vi "WaveformDataEventHandler Event Callback (CDB).vi"(4 "user event":refnum<user-event>, 5 "Event Data":cluster{"sender":refnum<k24>, "e":refnum<k24>}, 6 "Control Ref":refnum<k24>, 7 "Event Common Data":T1) -> ()   [LabVIEW 2020, in "NI_VS Waveform Streaming Interface.lvlib"]
uses:
  <vilib>/NI VeriStand/Execution/WaveformStreaming/NI_VS Waveform Streaming Interface.lvlib
  NationalInstruments.VeriStand.ClientAPI
  <vilib>/NI VeriStand/Execution/WaveformStreaming/Waveform Data Watcher Event Data (CDB).ctl
  <vilib>/NI VeriStand/Execution/WaveformStreaming/WaveformStreamSpecification.ctl
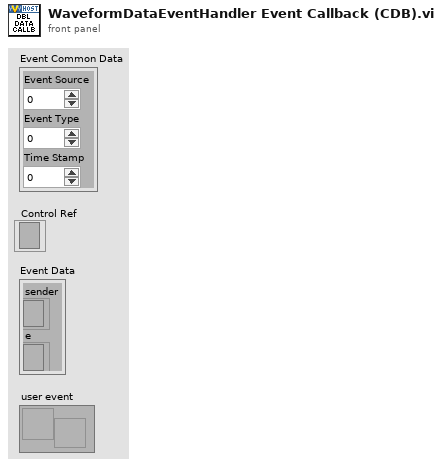
[diagram p1: front panel]
types:
  T1 = cluster{"Event Source":i32, "Event Type":u32, "Time Stamp":u32}
  T2 = typedef "NI_VS Waveform Streaming Interface.lvlib/Waveform Data Watcher Event Data (CDB).ctl" = cluster{"Data":cdb[], "dt":dbl, "offset from start (samples)":u64, "t0 at start":timestamp, "WaveformStreamSpecification":T3}
  T3 = typedef "NI_VS Waveform Streaming Interface.lvlib/WaveformStreamSpecification.ctl" = refnum<k24>
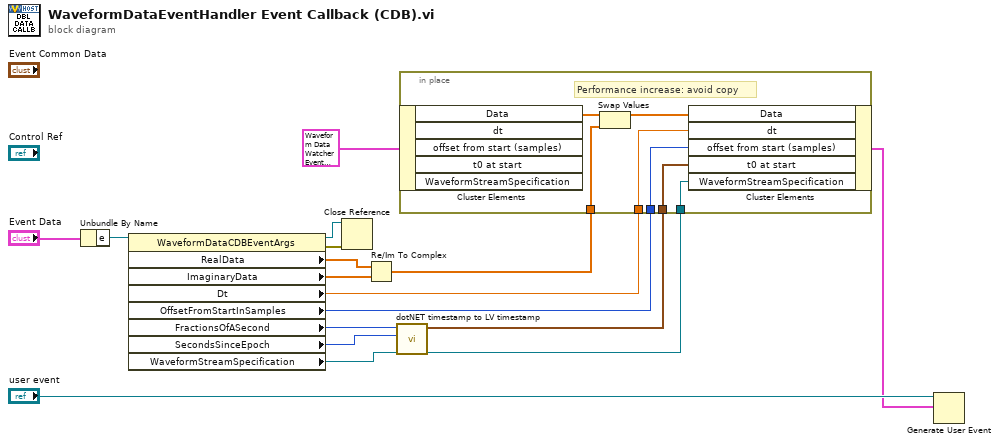
[diagram p0: block diagram]
diagram:
  n1 = Unbundle By Name("Event Data") -> ("e"=w14:refnum<k24>)
  n2 = property class="WaveformDataCDBEventArgs"(reference=w14) -> (reference out=w6:refnum<k24>, error out=w7:errorcluster, "RealData"=w5:dbl[], "ImaginaryData"=w4:dbl[], "Dt"=w12:dbl, "OffsetFromStartInSamples"=w11:u64, "FractionsOfASecond"=w2:u64, "SecondsSinceEpoch"=w1:i64, "WaveformStreamSpecification"=w9:refnum<k24>)  [unwired: 1 in]
  n3 = Close Reference(reference=w6, error in (no error)=w7) -> ()  [unwired: 1 out]
  n4 = Re/Im To Complex(1:w4, 2:w5) -> (0:w3:cdb[])
  n5 = call <vilib>:"dotNET timestamp to LV timestamp.vi"("seconds since epoch"=w1, "positive fractions of a second"=w2) -> ("t0"=w10:timestamp)  [unwired: 9 in]
  n6 = in-place {
    in-place-border: w3 -> [w22]
    in-place-border: w12 -> [w20]
    in-place-border: w11 -> [w19]
    in-place-border: w10 -> [w18]
    in-place-border: w9 -> [w17]
    # "Performance increase: avoid copy"
    n7 = in-place-cluster #1(T2 {"Data"=[], "dt"=0.0, "offset from start (samples)"=0, "t0 at start"=timestamp(0 s since 1904-01-01), "WaveformStreamSpecification"=refnum} ("event data")) -> ("Data"=w23:cdb[])  [unwired: 4 out]
    n8 = Swap Values(12:w23, 14:w22) -> (1:w21:cdb[])  [unwired: 1 in, 1 out]
    n9 = in-place-cluster #1("Data"=w21, "dt"=w20, "offset from start (samples)"=w19, "t0 at start"=w18, "WaveformStreamSpecification"=w17) -> (w8:T2)
  }
  n10 = Generate User Event(user event="user event", event data cluster=w8) -> ()  [unwired: 2 in, 2 out]
